vi "GUI Target Select.vi"(8 "error in":errorcluster, 10 "Control_Reference":refnum<vi>, 11 "SwitchMatrix in":refnum<class "SwitchMatrix.lvclass">) -> (0 "error out":errorcluster, 1 "Value":bool, 2 "Target":string, 3 "SwitchMatrix out":refnum<class "SwitchMatrix.lvclass">)   [LabVIEW 2019, in "SwitchMatrix.lvlib" / "SwitchMatrix.lvclass"]
uses:
  Library/SwitchMatrix.lvclass
  Library/SwitchMatrix.lvclass/SwitchMatrix.ctl
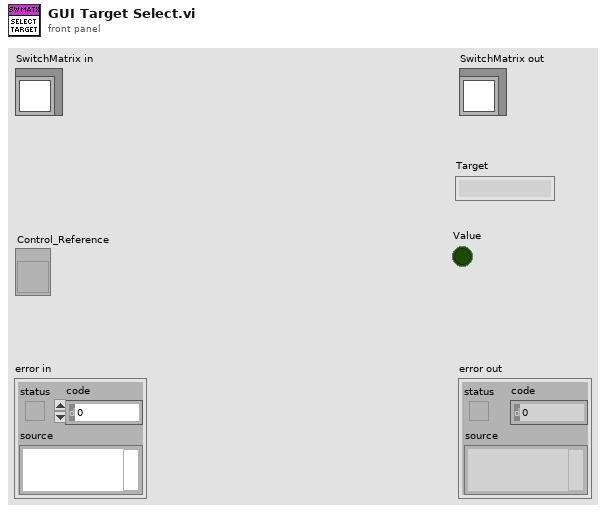
[diagram p1: front panel]
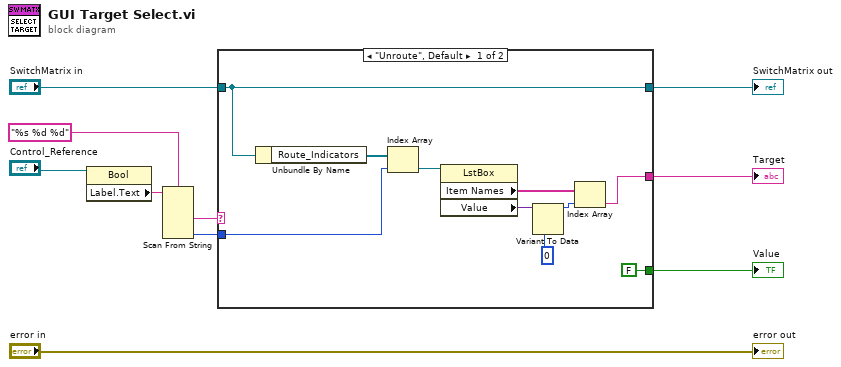
[diagram p0: block diagram]
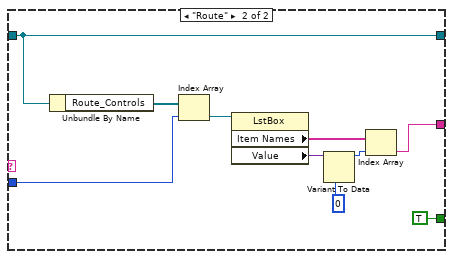
[diagram p2: hidden frame]
diagram:
  n1 = property class="Bool"(reference="Control_Reference") -> ("Label.Text"=w8:string)  [unwired: 1 in, 2 out]
  n2 = Scan From String(format string="%s %d %d", input string=w8) -> (output 1=w7:string, output 3=w5:i32)  [unwired: 6 in, 3 out]
  n3 = case shown="\"Unroute\", Default" w7 {
    tunnel: "SwitchMatrix in" -> [w20 w30]
    tunnel: w5 -> [w18 w28]
    tunnel: [FALSE TRUE] -> w4
    tunnel: [w20 w30] -> w3
    tunnel: [w12 w22] -> w2
    frame "Unroute", Default {
      n4 = Unbundle By Name(w20) -> ("Route_Indicators"=w19:refnum<vi>[])
      n5 = Index Array(array=w19, index=w18) -> (element=w13:refnum<vi>)
      n6 = property class="LstBox"(reference=w13) -> ("Item Names"=w14:string[], "Value"=w15:variant)  [unwired: 1 in, 2 out]
      n7 = Variant To Data(type=0, Variant=w15) -> (data=w16:i32)  [unwired: 1 in, 1 out]
      n8 = Index Array(array=w14, index=w16) -> (element=w12:string)
    }
    frame "Route" {
      n9 = Unbundle By Name(w30) -> ("Route_Controls"=w29:refnum<vi>[])
      n10 = Index Array(array=w29, index=w28) -> (element=w23:refnum<vi>)
      n11 = property class="LstBox"(reference=w23) -> ("Item Names"=w24:string[], "Value"=w25:variant)  [unwired: 1 in, 2 out]
      n12 = Variant To Data(type=0, Variant=w25) -> (data=w26:i32)  [unwired: 1 in, 1 out]
      n13 = Index Array(array=w24, index=w26) -> (element=w22:string)
    }
  }
  "SwitchMatrix out" <- w3
  "Target" <- w2
  "Value" <- w4
  "error out" <- "error in"
